vi "main - ONE Motor.vi"() -> ()   [LabVIEW 2018]
uses:
  Ctls/LoggingRate.ctl
  Ctls/MotorConfig.ctl
  Ctls/MotroConfigData.ctl
  Ctls/MagType.ctl
  Ctls/QueueData.ctl
  Ctls/State.ctl
  Ctls/CmdData.ctl
  Ctls/ConsumerLoopData.ctl
  Ctls/DisplayIndicator.ctl
  Ctls/DatabaseCmd.ctl
  Siemens S7 TCP v3_3 LV 8_5/Siemens S7 TCP v3_3 LV 8_5/S7 TCP API Library/S7 TCP.lvlib
panel:
  out "error out":errorcluster
  out "Motor#1_EmoStop?":bool caption="急停指示"
  in  "Speed Setting Checked?_4":bool
  in  "Speed Setting Checked?_3":bool
  in  "Speed Setting Checked?_2":bool
  in  "Speed Setting Checked?_1":bool
  in  "Motor_SpeedSetting#4":dbl caption="电机速度设定 1" min=0.0 max=50.0 format="%.3f"
  in  "Motor_SpeedSetting#3":dbl caption="电机速度设定 1" min=0.0 max=50.0 format="%.3f"
  in  "Motor_SpeedSetting#2":dbl caption="电机速度设定 1" min=0.0 max=50.0 format="%.3f"
  out "Motor#1_Speed":sgl(knob) caption="电机转速RPS" scale=0.01..50.0 scale format="%#.3f"
  out "Motor#1_ConfigData":T1 caption="电机配置数据"
  in  "Motor#1_Config":T2 caption="电机配置"
  in  "Motor#1_SpeedSet?":bool
  in  "Log Length":i32=50
  in  "Logging Rate":T4=enum."5Hz"
  in  "sample interval (ms)":i32=50
  in  "Record":bool
  out "Speed Log to Display":string[][](table)
  out "Data Read":u8[][](array[numeric])
  out "Float Data Valid?":bool[](array[boolean])
  out "Bool Data Valid":bool
  in  "Stop Button":bool
  out "SpeedCurve":sgl(graph) caption="实时显示"
  in  "ClearFault?":bool caption="故障复位"
  out "Motor#1_Fault?":bool caption="故障指示 1"
  out "Motor#1_Running?":bool caption="电机运行指示"
  out "Motor#1_Connected？":bool caption="远程允许"
  out "Motor#1_Current":dbl caption="电机电流   1" format="%1.2f"
  in  "Motor_SpeedSetting#1":dbl caption="电机速度设定 1" min=0.0 max=50.0 format="%.3f"
  in  "Motor#1_Start?":bool caption="电机启动   1"
  in  "Motor#1_Direction":bool caption="电机方向\n正转          反转    1"
  # "1#大电机"
  # "RPS"
  # "RPS"
  # "RPS"
  # "RPS"
  # "A"
  # "注意：切换励磁请手动更改驱动器参数P50082,\n 当P50082=0时为永磁，P50082=1时为励磁！！"
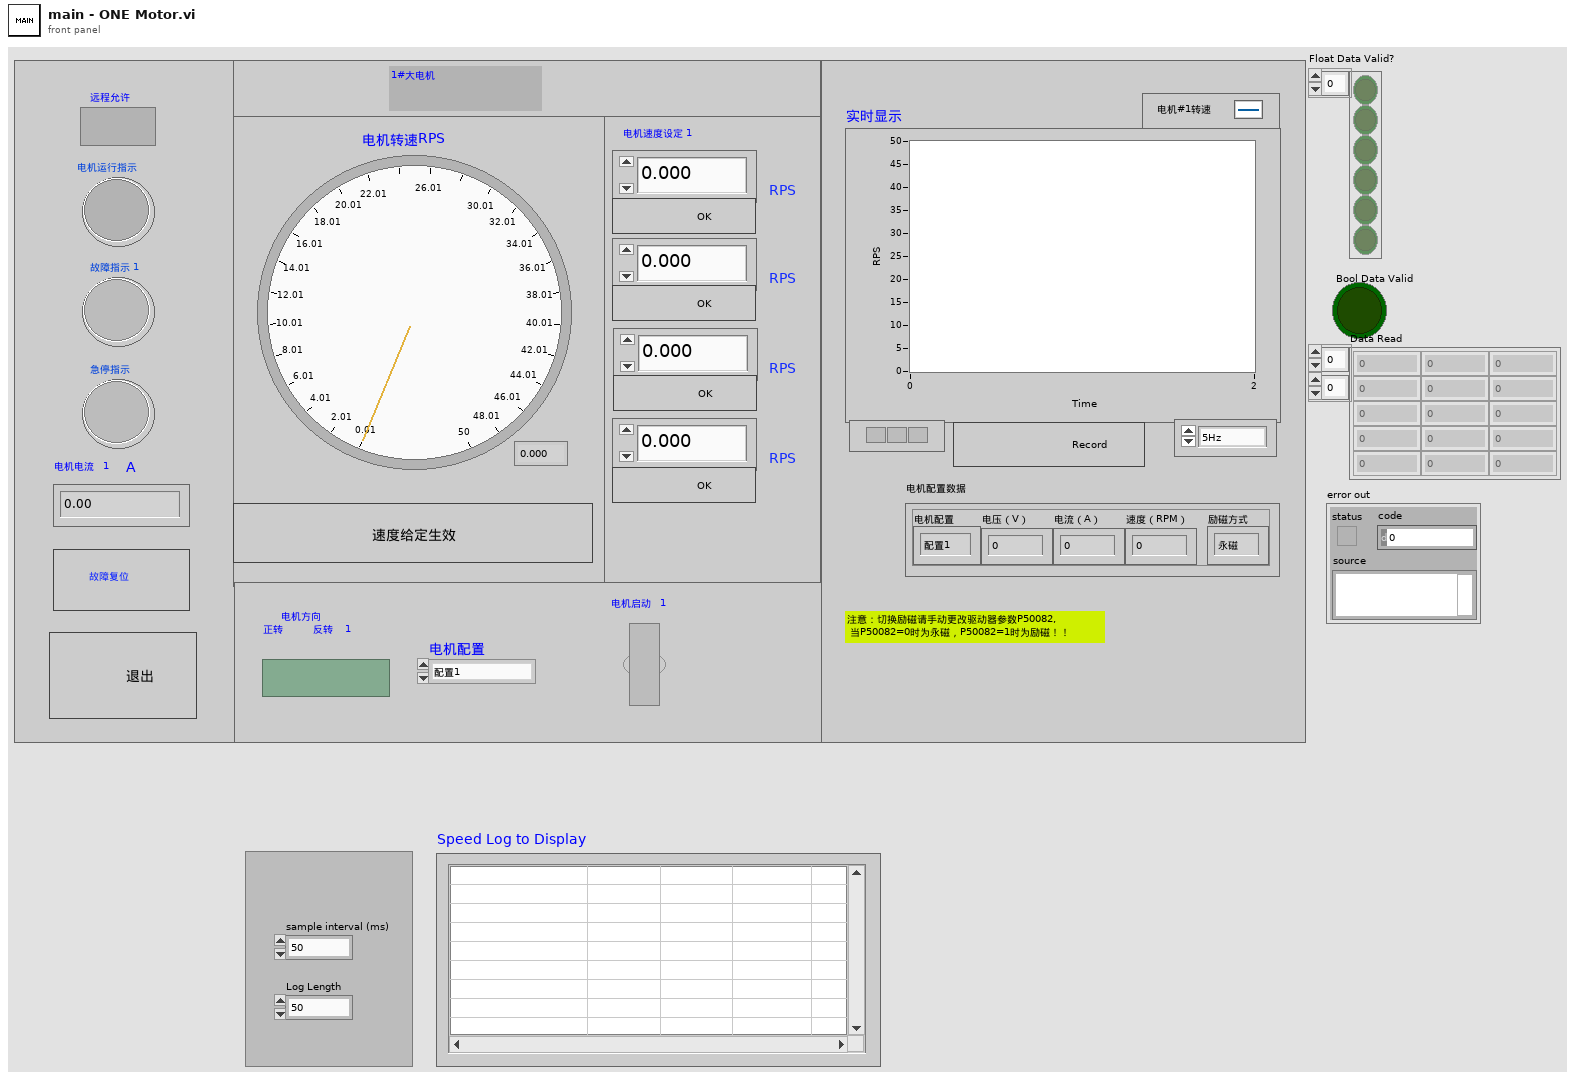
[diagram p1: front panel]
types:
  T1 = typedef "MotroConfigData.ctl" = cluster{"电机配置":T2, "电压（V）":dbl, "电流（A）":dbl, "速度（RPM）":dbl, "励磁方式":T3}
  T2 = typedef "MotorConfig.ctl" = enum16{"配置1", "配置2", "配置3", "配置4"}
  T3 = typedef "MagType.ctl" = enum16{"永磁", "励磁"}
  T4 = typedef "LoggingRate.ctl" = enum16{"1Hz", "2Hz", "5Hz", "10Hz", "20Hz"}
  T5 = typedef "ConsumerLoopData.ctl" = cluster{"CmdU16":u16, "Log File Path":path, "PLC Data":T6, "TCP Connection Ref":refnum<k5>, "Config File Path":path}
  T6 = typedef "DisplayIndicator.ctl" = cluster{"CommConnected_1":bool, "Run_1?":bool, "Fault_1?":bool, "CommConnected_2":bool, "Run_2?":bool, "Fault_2?":bool, "Motor Speed 2":sgl, "Motor Speed_1":sgl, "Motor Current_1":sgl, "Motor Current_2":sgl, "Motor1ConfigData":T1, "Motor2ConfigData":T1, "EmoStop_1?":bool}
  T7 = typedef "State.ctl" = enum16{"poll data command", "display update", "init", "send bool command", "send float command", "datalog", "error", "fix rating rpm 1", "fix rating rpm 2", "fix both rating rpm", "fix rating rpm all", "terminate", "log Motor Speed Setting"}
  T8 = typedef "QueueData.ctl" = cluster{"State":T7, "Command Data":T9}
  T9 = typedef "CmdData.ctl" = cluster{"Address Areas":u8, "Data Block #":u16, "Start Address (bytes)":u32, "Write Data Float":sgl, "Bit #":u16, "Write Data Boolean":bool}
  T10 = typedef "DatabaseCmd.ctl" = enum16{"Insert Table Title", "Add One Record", "Delete Record", "Get Table Records", "Clear"}
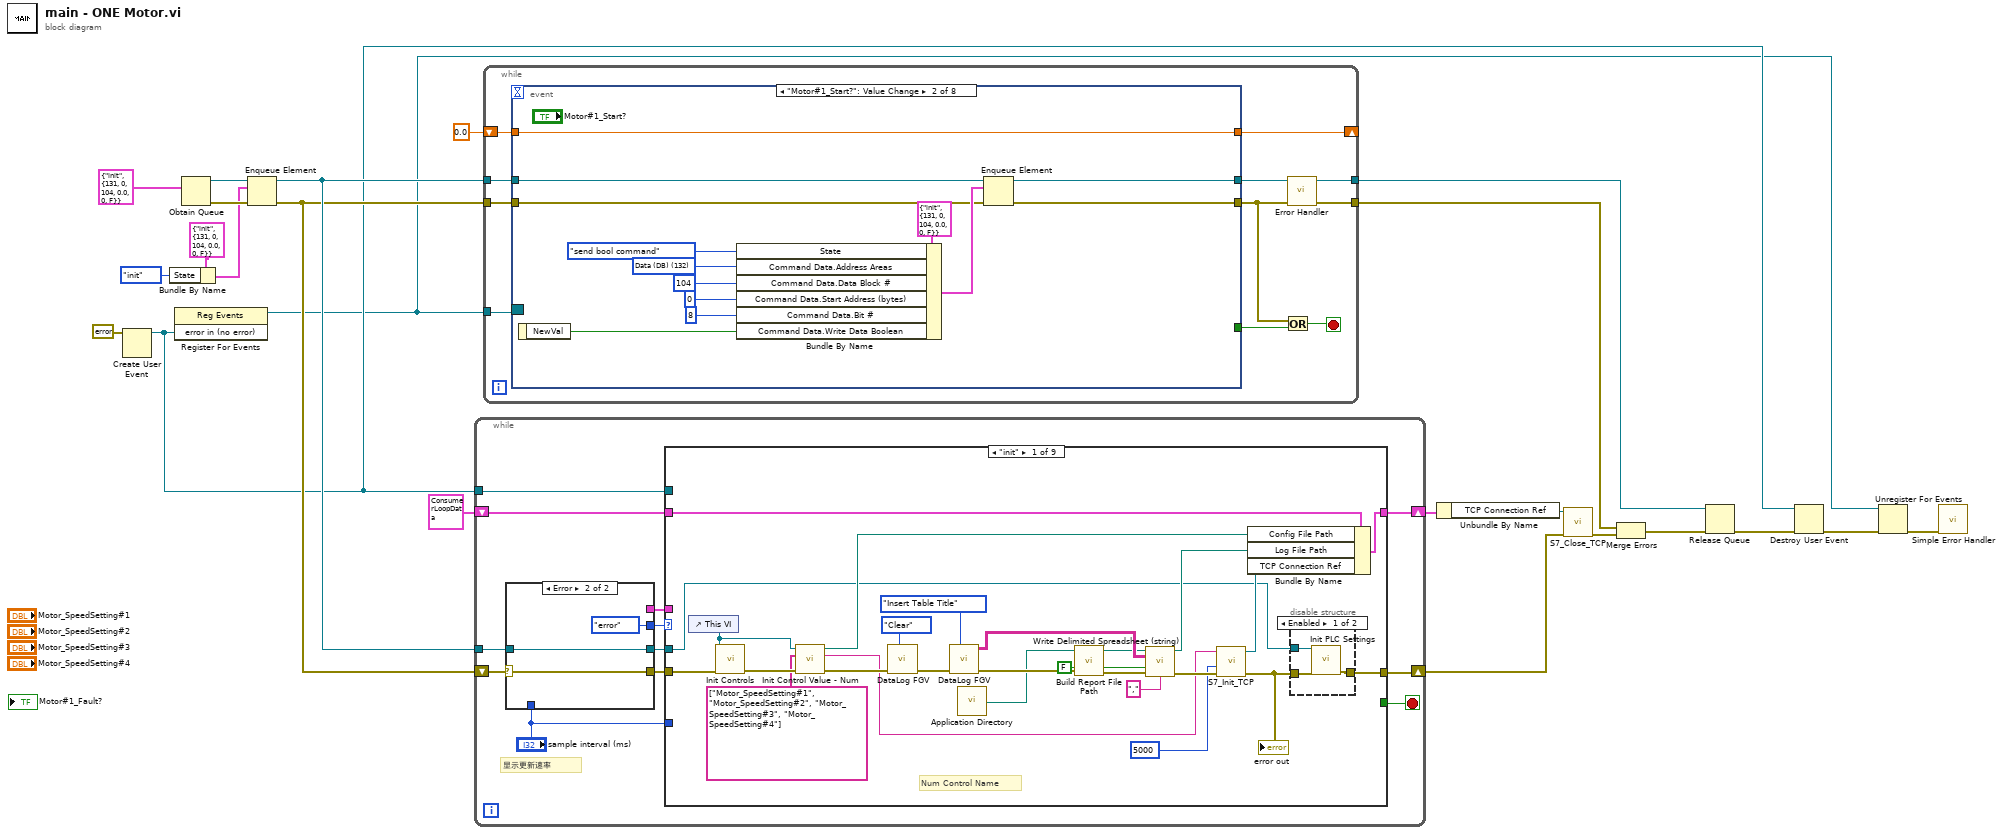
[diagram p0: block diagram]
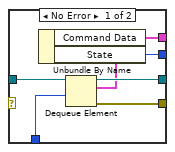
[diagram p2: hidden frame]
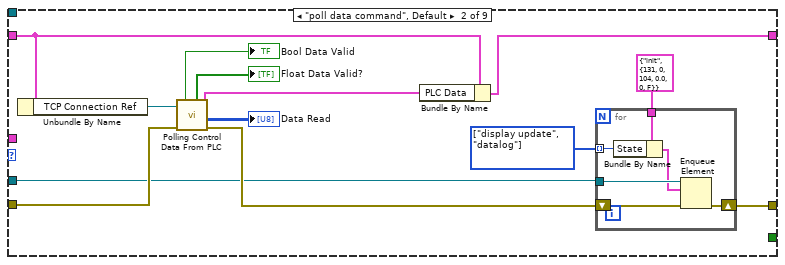
[diagram p4: hidden frame]
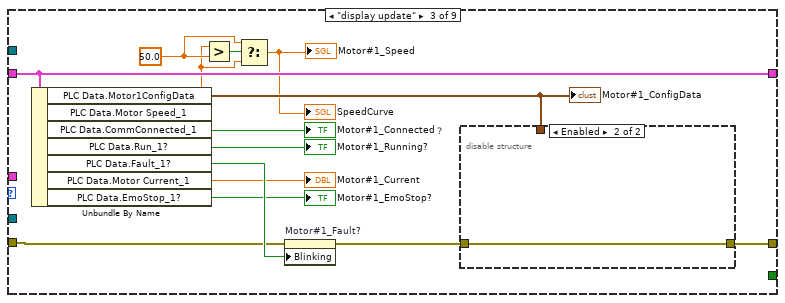
[diagram p5: hidden frame]
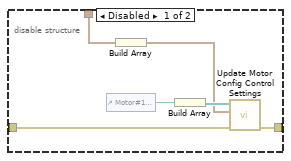
[diagram p6: hidden frame]
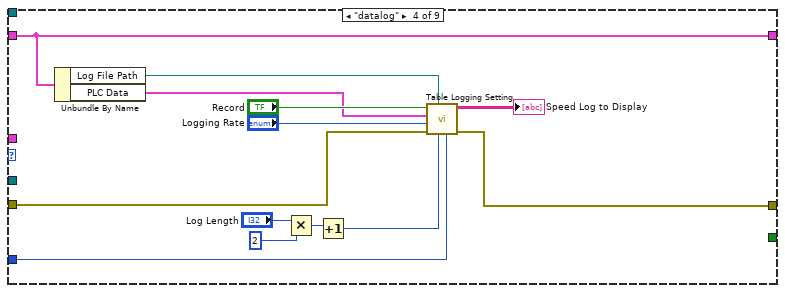
[diagram p7: hidden frame]
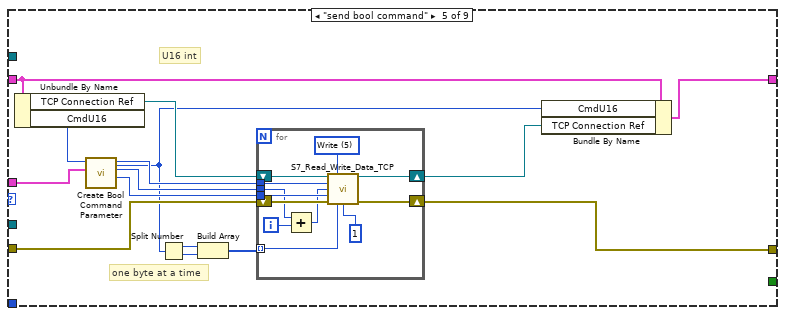
[diagram p8: hidden frame]
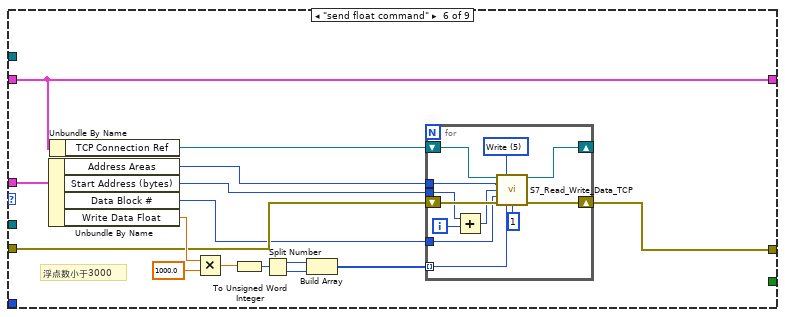
[diagram p9: hidden frame]
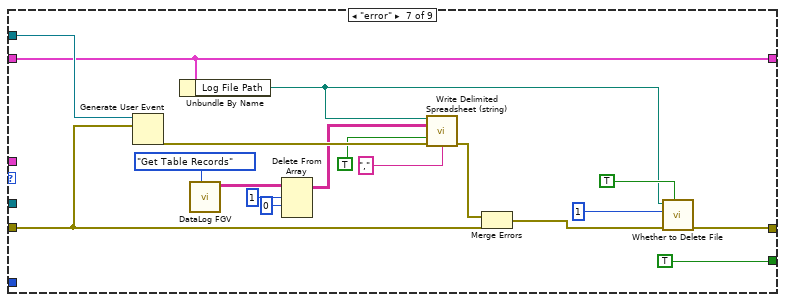
[diagram p10: hidden frame]
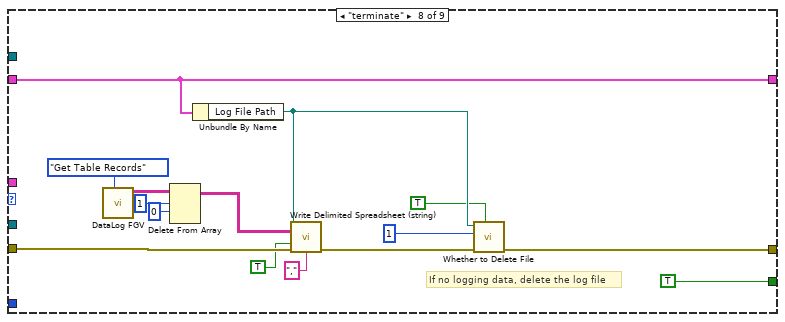
[diagram p11: hidden frame]
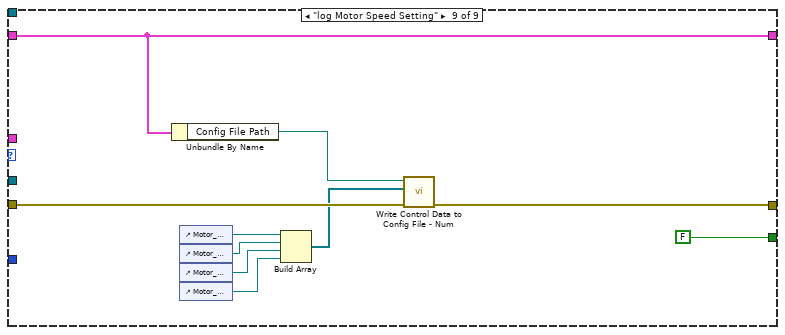
[diagram p12: hidden frame]
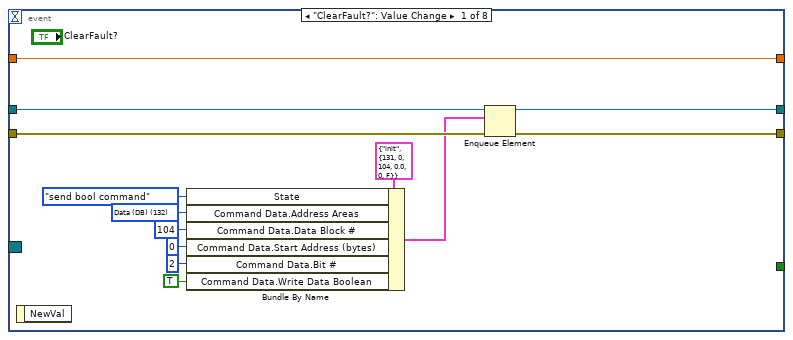
[diagram p13: hidden frame]
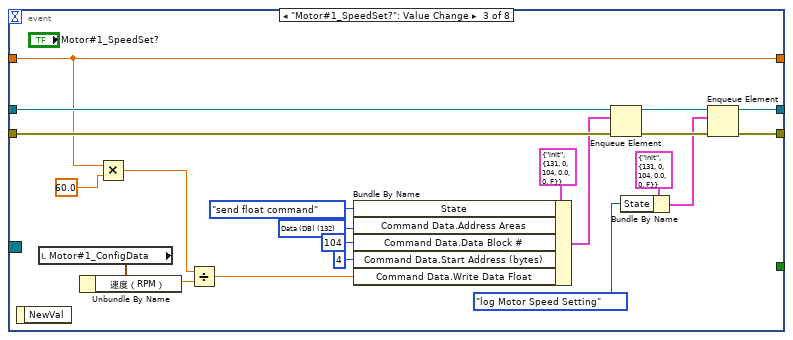
[diagram p14: hidden frame]
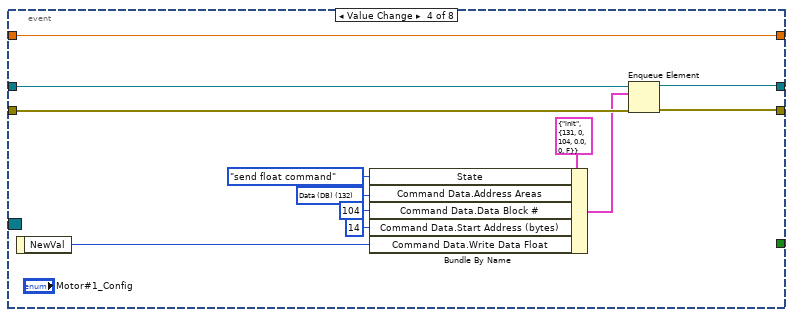
[diagram p15: hidden frame]
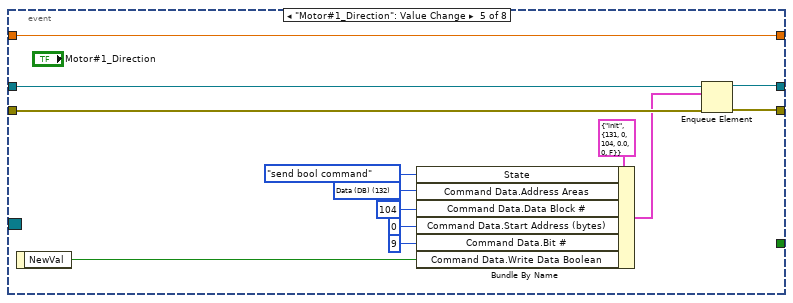
[diagram p16: hidden frame]
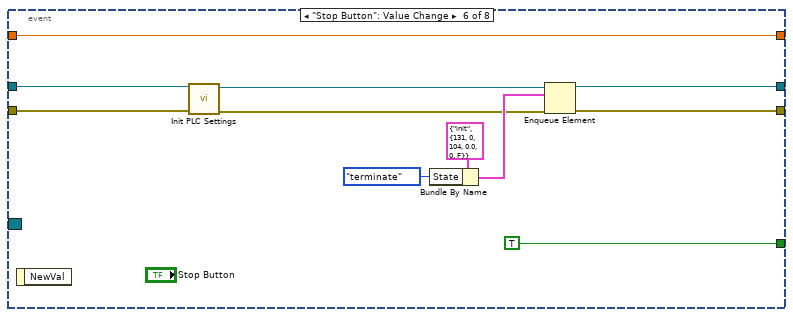
[diagram p17: hidden frame]
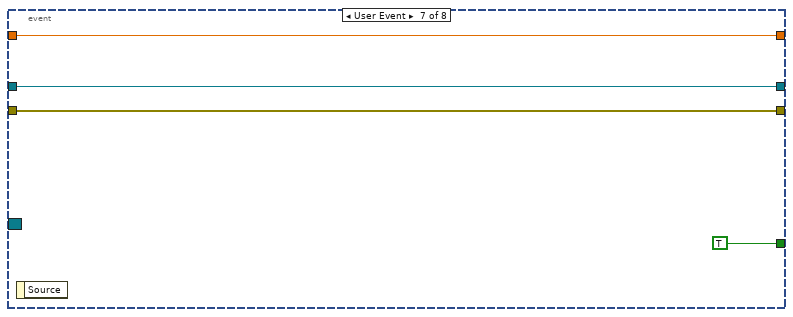
[diagram p18: hidden frame]
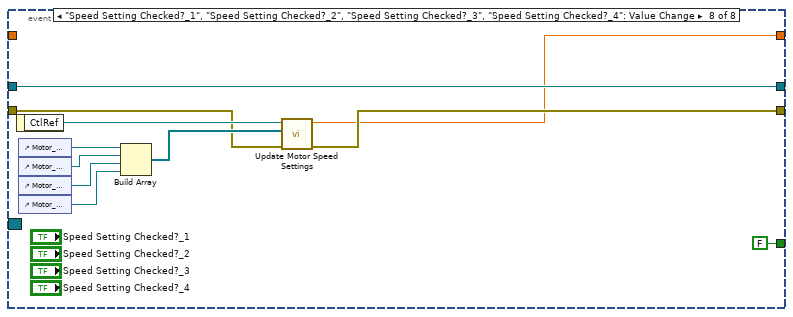
[diagram p19: hidden frame]
diagram:
  n1 = Create User Event(user event datatype=errorcluster {"status"=FALSE, "code"=0, "source"=""} ("error in (no error)")) -> (user event=w14:refnum<user-event>)  [unwired: 1 in, 1 out]
  n2 = Bundle By Name(cluster=T8 {"State"=enum."init", "Command Data"={"Address Areas"=131, "Data Block #"=0, "Start Address (bytes)"=104, "Write Data Float"=0.0, "Bit #"=0, "Write Data Boolean"=FALSE}} ("element"), "State"=State."init") -> (w16:T8)
  n3 = register-events(w14) -> (reference out=w12:refnum<event-registration>)  [unwired: 2 in, 1 out]
  n4 = Obtain Queue(element data type=T8 {"State"=enum."init", "Command Data"={"Address Areas"=131, "Data Block #"=0, "Start Address (bytes)"=104, "Write Data Float"=0.0, "Bit #"=0, "Write Data Boolean"=FALSE}} ("QData")) -> (queue out=w22:refnum<queue>, error out=w20:errorcluster)  [unwired: 4 in, 1 out]
  n5 = Enqueue Element(queue=w22, element=w16, error in (no error)=w20) -> (queue out=w21:refnum<queue>, error out=w19:errorcluster)  [unwired: 1 in, 1 out]
  n6 = while {
    tunnel: w21 -> [w27]
    tunnel: w14 -> [w30]
    shift-right: [w28] -> w11
    shift-left: w19 -> [w29]
    shift-right: [w25] -> w9
    shift-left: T5 {"CmdU16"=0, "Log File Path"=path "", "PLC Data"={"CommConnected_1"=FALSE, "Run_1?"=FALSE, "Fault_1?"=FALSE, "CommConnected_2"=FALSE, "Run_2?"=FALSE, "Fault_2?"=FALSE, "Motor Speed 2"=0.0, "Motor Speed_1"=0.0, "Motor Current_1"=0.0, "Motor Current_2"=0.0, "Motor1ConfigData"={"电机配置"=enum."配置1", "电压（V）"=0.0, "电流（A）"=0.0, "速度（RPM）"=0.0, "励磁方式"=enum."永磁"}, "Motor2ConfigData"={"电机配置"=enum."配置1", "电压（V）"=0.0, "电流（A）"=0.0, "速度（RPM）"=0.0, "励磁方式"=enum."永磁"}, "EmoStop_1?"=FALSE}, "TCP Connection Ref"=refnum, "Config File Path"=path ""} ("Consumer Loop Data") -> [w26]
    stop <- w31 stop-if-true
    # "显示更新速率"
    n7 = case shown="Error" w29 {
      selector: w29 -> [_ w45]
      tunnel: [w42 w44] -> w35
      tunnel: [w41 w45] -> w34
      tunnel: [w39 State."error" ("State")] -> w33
      tunnel: [w38 _] -> w32
      tunnel: w27 -> [w37 w44]
      tunnel: "sample interval (ms)" -> [w36 _]
      frame No Error {
        n8 = Dequeue Element(queue=w37, timeout in ms (-1)=w36) -> (queue out=w42:refnum<queue>, element=w40:T8, error out=w41:errorcluster)  [unwired: 1 in, 1 out]
        n9 = Unbundle By Name(w40) -> ("Command Data"=w38:T9, "State"=w39:T7)
      }
      frame Error {
      }
    }
    n10 = case shown="\"init\"" w33 {
      tunnel: w35 -> [w47 w85 _ _ _ _ _ _ _]
      tunnel: w34 -> [w57 w88 w105 w126 w143 w164 w198 w210 w223]
      tunnel: [w58 w86 w108 w125 w135 w158 w184 w204 w217] -> w28
      tunnel: w32 -> [_ _ _ _ w142 w170 _ _ _]
      tunnel: [_ _ _ _ _ _ TRUE ("Data Valid") TRUE ("Data Valid") FALSE ("Data Valid")] -> w31
      tunnel: w30 -> [_ _ _ _ _ _ w199 _ _]
      tunnel: w26 -> [w56 w82 w107 w117 w132 w156 w188 w206 w225]
      tunnel: [w55 w80 w107 w117 w129 w156 w188 w206 w225] -> w25
      tunnel: "sample interval (ms)" -> [_ _ _ w116 _ _ _ _ _]
      frame "init" {
        # "Num Control Name"
        n11 = control-ref of="This VI"() -> (w48:refnum<vi>)
        n12 = call "Init Controls.vi"("error in"=w57, "VI ref"=w48) -> ("error out"=w54:errorcluster)  [unwired: 9 in]
        n13 = call "Init Control Value - Num.vi"("error in (no error)"=w54, "Num Control Names"=string[] ["Motor_SpeedSetting#1", "Motor_SpeedSetting#2", "Motor_SpeedSetting#3", "Motor_SpeedSetting#4"], "This VI"=w48) -> ("error out"=w53:errorcluster, "PLC IP"=w46:string, "Config File Path"=w50:path)  [unwired: 6 in]
        n14 = call "DataLog FGV.vi"("Method"=DatabaseCmd."Clear", "error in (no error)"=w53) -> ("error out"=w71:errorcluster)  [unwired: 7 in, 2 out]
        n15 = call "DataLog FGV.vi"("Method"=DatabaseCmd."Insert Table Title", "error in (no error)"=w71) -> ("error out"=w70:errorcluster, "Speed Log"=w69:string[][])  [unwired: 7 in, 1 out]
        n16 = call <vilib>:"Application Directory.vi"() -> ("Application Directory"=w63:path)
        n17 = call "Build Report File Path.vi"("error in (no error)"=w70, "File Path in"=w63) -> ("error out"=w67:errorcluster, "Report Path out"=w68:path)  [unwired: 8 in]
        n18 = call "Write Delimited Spreadsheet (string).vi"("Path"=w68, "2D data"=w69, "append to file?"=FALSE ("append to file? (new file:F)"), "error in"=w67, "delimiter (\\t)"="," ("delimiter (\\t)")) -> ("path"=w51:path, "error out"=w61:errorcluster)  [unwired: 9 in]
        n19 = call "S7_Init_TCP.vi"("error in"=w61, "Connection Timeout"=u32 5000, "IP Address"=w46) -> ("error out"=w59:errorcluster, "TCP Connection Ref"=w52:refnum<k5>)  [unwired: 2 in, 5 out]
        "error out" <- w59
        n20 = Bundle By Name(cluster=w56, "Config File Path"=w50, "Log File Path"=w51, "TCP Connection Ref"=w52) -> (w55:T5)
        n21 = disable-structure shown="Enabled" {
          disable-tunnel: w59 -> [w74 w75]
          disable-tunnel: [w73 w75] -> w58
          disable-tunnel: w47 -> [w72 _]
          frame Enabled {
            n22 = call "Init PLC Settings.vi"("error in"=w74, "queue in"=w72) -> ("error out"=w73:errorcluster)  [unwired: 8 in, 1 out]
          }
          frame Disabled {
          }
        }
      }
      frame "poll data command", Default {
        w83 = T7[] [enum."display update", enum."datalog"] items=["poll data command", "display update", "init", "send bool command", "send float command", "datalog", "error", "fix rating rpm 1", "fix rating rpm 2", "fix both rating rpm", "fix rating rpm all", "terminate", "log Motor Speed Setting"]
        n23 = Unbundle By Name(w82) -> ("TCP Connection Ref"=w79:refnum<k5>)
        n24 = call "Polling Control Data From PLC.vi"("error in (no error)"=w88, "TCP Network Connection in"=w79) -> ("error out"=w87:errorcluster, "Data Read"=→"Data Read":u8[][], "PLC Data out"=w81:T6, "Bool Data Valid"=→"Bool Data Valid":bool, "Float Data Valid?"=→"Float Data Valid?":bool[])  [unwired: 2 in, 3 out]
        n25 = Bundle By Name(cluster=w82, "PLC Data"=w81) -> (w80:T5)
        n26 = for {
          tunnel: w85 -> [w92]
          shift-right: [w93] -> w86
          shift-left: w87 -> [w94]
          tunnel: T8 {"State"=enum."init", "Command Data"={"Address Areas"=131, "Data Block #"=0, "Start Address (bytes)"=104, "Write Data Float"=0.0, "Bit #"=0, "Write Data Boolean"=FALSE}} ("QData") -> [w90]
          tunnel: w83 -> [w89] mode=indexing
          n27 = Bundle By Name(cluster=w90, "State"=w89) -> (w91:T8)
          n28 = Enqueue Element(queue=w92, element=w91, error in (no error)=w94) -> (error out=w93:errorcluster)  [unwired: 1 in, 2 out]
        }
      }
      frame "display update" {
        w98 = sgl 50.0 ("y")
        n29 = Unbundle By Name(w107) -> ("PLC Data.Motor1ConfigData"=w100:T1, "PLC Data.Motor Speed_1"=w97:sgl, "PLC Data.CommConnected_1"=→"Motor#1_Connected？":bool, "PLC Data.Run_1?"=→"Motor#1_Running?":bool, "PLC Data.Fault_1?"=w106:bool, "PLC Data.Motor Current_1"=→"Motor#1_Current":sgl, "PLC Data.EmoStop_1?"=→"Motor#1_EmoStop?":bool)
        "Motor#1_ConfigData" <- w100
        n30 = Greater?(x=w97, y=w98) -> (0:w99:bool)
        n31 = Select(t=w98, s=w99, f=w97) -> (s? t:f=→"SpeedCurve" →"Motor#1_Speed":sgl)
        n32 = property on="Motor#1_Fault?" class="Bool (strict)"(error in=w105, "Blinking"=w106) -> (error out=w101:errorcluster)  [unwired: 1 in, 1 out]
        n33 = disable-structure shown="Enabled" {
          disable-tunnel: [w114 w115] -> w108
          disable-tunnel: w101 -> [w113 w115]
          disable-tunnel: w100 -> [w110 _]
          frame Disabled {
            n34 = control-ref of="Motor#1_Config"() -> (w112:refnum<vi>)
            n35 = Build Array(w110) -> (w109:T1[])
            n36 = Build Array(w112) -> (w111:refnum<vi>[])
            n37 = call "Update Motor Config Control Settings.vi"("error in (no error)"=w113, "Motor Config Data"=w109, "Motor Config Refs"=w111) -> ("error out"=w114:errorcluster)  [unwired: 8 in]
          }
          frame Enabled {
          }
        }
      }
      frame "datalog" {
        n38 = Unbundle By Name(w117) -> ("Log File Path"=w119:path, "PLC Data"=w118:T6)
        n39 = Multiply(x="Log Length", y=2) -> (x*y=w121:i32)
        n40 = Increment(x=w121) -> (x+1=w120:i32)
        n41 = call "Table Logging Setting.vi"("sample interval (ms)"=w116, "Log Length"=w120, "Log File path"=w119, "error in (no error)"=w126, "Logging Rate"="Logging Rate", "Data In"=w118, "Record"="Record") -> ("error out"=w125:errorcluster, "Speed Log to Display"=→"Speed Log to Display":string[][])  [unwired: 3 in]
      }
      frame "send bool command" {
        # "one byte at a time"
        # "U16 int"
        n42 = Unbundle By Name(w132) -> ("TCP Connection Ref"=w133:refnum<k5>, "CmdU16"=w134:u16)
        n43 = call "Create Bool Command Parameter.vi"("Command Data"=w142, "Cmd U16"=w134) -> ("Data Block #"=w139:u16, "Start Address (bytes)"=w140:u32, "Address Areas"=w141:u8, "Cmd U16 out"=w131:u16)  [unwired: 6 in]
        n44 = Split Number(x=w131) -> (hi(x)=w137:u8, lo(x)=w136:u8)
        n45 = Build Array(w137, w136) -> (w138:u8[])
        n46 = for {
          tunnel: w141 -> [w151]
          tunnel: w140 -> [w145]
          tunnel: w139 -> [w150]
          shift-right: [w152] -> w130
          shift-left: w133 -> [w155]
          shift-right: [w148] -> w135
          shift-left: w143 -> [w154]
          tunnel: w138 -> [w147] mode=indexing
          i -> [w146]
          w153 = u8 5 items=["Read"=4, "Write"=5] ("Read / Write")
          n47 = Add(x=w145, y=w146) -> (x+y=w144:u32)
          n48 = call "S7_Read_Write_Data_TCP.vi"("TCP Connection Ref"=w155, "Read / Write"=w153, "Address Areas"=w151, "Start Address (bytes)"=w144, "Data Block #"=w150, "error in"=w154, "Write Data"=w147, "Length (bytes)"=u16 1) -> ("TCP Connection Ref Out"=w152:refnum<k5>, "error out"=w148:errorcluster)  [unwired: 2 in, 4 out]
        }
        n49 = Bundle By Name(cluster=w132, "CmdU16"=w131, "TCP Connection Ref"=w130) -> (w129:T5)
      }
      frame "send float command" {
        # "浮点数小于3000"
        n50 = Unbundle By Name(w170) -> ("Address Areas"=w163:u8, "Start Address (bytes)"=w162:u32, "Data Block #"=w161:u16, "Write Data Float"=w169:sgl)
        n51 = Unbundle By Name(w156) -> ("TCP Connection Ref"=w157:refnum<k5>)
        n52 = Multiply(x=w169, y=sgl 1000.0) -> (x*y=w167:sgl)
        n53 = To Unsigned Word Integer(number=w167) -> (unsigned 16bit integer=w166:u16)
        n54 = Split Number(x=w166) -> (hi(x)=w160:u8, lo(x)=w159:u8)
        n55 = Build Array(w160, w159) -> (w165:u8[])
        n56 = for {
          shift-right: [w179] -> _
          shift-left: w157 -> [w182]
          shift-right: [w177] -> w158
          shift-left: w164 -> [w181]
          tunnel: w165 -> [w174] mode=indexing
          tunnel: w163 -> [w173]
          tunnel: w162 -> [w172]
          tunnel: w161 -> [w171]
          i -> [w176]
          w180 = u8 5 items=["Read"=4, "Write"=5] ("Read / Write")
          n57 = Add(x=w172, y=w176) -> (x+y=w175:u32)
          n58 = call "S7_Read_Write_Data_TCP.vi"("TCP Connection Ref"=w182, "Read / Write"=w180, "Address Areas"=w173, "Start Address (bytes)"=w175, "Data Block #"=w171, "error in"=w181, "Write Data"=w174, "Length (bytes)"=u16 1) -> ("TCP Connection Ref Out"=w179:refnum<k5>, "error out"=w177:errorcluster)  [unwired: 2 in, 4 out]
        }
      }
      frame "error" {
        n59 = Generate User Event(user event=w199, event data cluster=w198) -> (error out=w197:errorcluster)  [unwired: 2 in, 1 out]
        n60 = Unbundle By Name(w188) -> ("Log File Path"=w183:path)
        n61 = call "DataLog FGV.vi"("Method"=DatabaseCmd."Get Table Records") -> ("Speed Log"=w193:string[][])  [unwired: 8 in, 2 out]
        n62 = Delete From Array(array=w193, length=1, index (row)=0) -> (array with subset deleted=w190:string[][])  [unwired: 1 in, 1 out]
        n63 = call "Write Delimited Spreadsheet (string).vi"("Path"=w183, "2D data"=w190, "append to file?"=TRUE ("append to file? (new file:F)"), "error in"=w197, "delimiter (\\t)"="," ("delimiter (\\t)")) -> ("error out"=w196:errorcluster)  [unwired: 9 in, 1 out]
        n64 = Merge Errors(w196, w198) -> (w185:errorcluster)
        n65 = call "Whether to Delete File.vi"("Del Log file?"=TRUE, "error in (no error)"=w185, "Number of lines"=1, "File path"=w183) -> ("error out"=w184:errorcluster)  [unwired: 7 in]
      }
      frame "terminate" {
        # "If no logging data, delete the log file"
        n66 = call "DataLog FGV.vi"("Method"=DatabaseCmd."Get Table Records") -> ("Speed Log"=w213:string[][])  [unwired: 8 in, 2 out]
        n67 = Delete From Array(array=w213, length=1, index (row)=0) -> (array with subset deleted=w209:string[][])  [unwired: 1 in, 1 out]
        n68 = Unbundle By Name(w206) -> ("Log File Path"=w203:path)
        n69 = call "Write Delimited Spreadsheet (string).vi"("Path"=w203, "2D data"=w209, "append to file?"=TRUE ("append to file? (new file:F)"), "error in"=w210, "delimiter (\\t)"="," ("delimiter (\\t)")) -> ("error out"=w205:errorcluster)  [unwired: 9 in, 1 out]
        n70 = call "Whether to Delete File.vi"("Del Log file?"=TRUE, "error in (no error)"=w205, "Number of lines"=1, "File path"=w203) -> ("error out"=w204:errorcluster)  [unwired: 7 in]
      }
      frame "log Motor Speed Setting" {
        n71 = Unbundle By Name(w225) -> ("Config File Path"=w224:path)
        n72 = control-ref of="Motor_SpeedSetting#1"() -> (w222:refnum<vi>)
        n73 = control-ref of="Motor_SpeedSetting#2"() -> (w221:refnum<vi>)
        n74 = control-ref of="Motor_SpeedSetting#3"() -> (w220:refnum<vi>)
        n75 = control-ref of="Motor_SpeedSetting#4"() -> (w219:refnum<vi>)
        n76 = Build Array(w222, w221, w220, w219) -> (w218:refnum<vi>[])
        n77 = call "Write Control Data to Config File - Num.vi"("error in (no error)"=w223, "Num Controls"=w218, "Config File Path"=w224) -> ("error out"=w217:errorcluster)  [unwired: 8 in]
      }
    }
  }
  n78 = while {
    tunnel: w21 -> [w236]
    tunnel: w19 -> [w235]
    tunnel: w12 -> [w234]
    tunnel: [w229] -> w6
    tunnel: [w228] -> w5
    shift-right: [w227] -> _
    shift-left: 0.0 ("Motor Speed") -> [w226]
    stop <- w232 stop-if-true
    n79 = event shown="[1] \"Motor#1_Start?\": Value Change" {
      selector: w234 -> [_ _ _ _ _ _ _ _]
      dyn-events: _ -> [_ _ _ _ _ _ _ _]
      timeout: _ -> [_ _ _ _ _ _ _ _]
      tunnel: [_ _ _ _ _ TRUE ("Stop Button") TRUE ("Stop Button") FALSE ("Stop Button")] -> w233
      tunnel: w236 -> [w249 w259 w282 w294 w307 w313 w323 w328]
      tunnel: w235 -> [w248 w258 w281 w292 w305 w311 w322 w327]
      tunnel: [w244 w251 w269 w293 w306 w318 w323 w328] -> w231
      tunnel: [w245 w250 w264 w291 w304 w317 w322 w326] -> w230
      tunnel: [w237 w252 w263 w284 w296 w309 w320 w324] -> w227
      tunnel: w226 -> [w237 w252 w263 w284 w296 w309 w320 _]
      event "ClearFault?": Value Change {
        w242 = u8 132 items=["I/O (P)"=128, "Input (I)"=129, "Output (Q)"=130, "Bit Memory (M)"=131, "Data (DB)"=132, "Instance Data (DI)"=133, "Local Data (L)"=134, "Predecessor Local Data (VL)"=135] ("Address Areas")
        n80 = event-data() -> ()  [unwired: 1 in, 1 out]
        n81 = Bundle By Name(cluster=T8 {"State"=enum."init", "Command Data"={"Address Areas"=131, "Data Block #"=0, "Start Address (bytes)"=104, "Write Data Float"=0.0, "Bit #"=0, "Write Data Boolean"=FALSE}} ("QData"), "State"=State."send bool command", "Command Data.Address Areas"=w242, "Command Data.Data Block #"=u16 104 ("Data Block #"), "Command Data.Start Address (bytes)"=u32 0 ("Start Address (bytes)"), "Command Data.Bit #"=u16 2 ("Bit #"), "Command Data.Write Data Boolean"=TRUE ("Write Data Boolean")) -> (w247:T8)
        n82 = Enqueue Element(queue=w249, element=w247, error in (no error)=w248) -> (queue out=w244:refnum<queue>, error out=w245:errorcluster)  [unwired: 1 in, 1 out]
      }
      event "Motor#1_Start?": Value Change {
        w257 = u8 132 items=["I/O (P)"=128, "Input (I)"=129, "Output (Q)"=130, "Bit Memory (M)"=131, "Data (DB)"=132, "Instance Data (DI)"=133, "Local Data (L)"=134, "Predecessor Local Data (VL)"=135] ("Address Areas")
        n83 = event-data() -> ("NewVal"=w253:bool)  [unwired: 1 in]
        n84 = Bundle By Name(cluster=T8 {"State"=enum."init", "Command Data"={"Address Areas"=131, "Data Block #"=0, "Start Address (bytes)"=104, "Write Data Float"=0.0, "Bit #"=0, "Write Data Boolean"=FALSE}} ("QData"), "State"=State."send bool command", "Command Data.Address Areas"=w257, "Command Data.Data Block #"=u16 104 ("Data Block #"), "Command Data.Start Address (bytes)"=u32 0 ("Start Address (bytes)"), "Command Data.Bit #"=u16 8 ("Bit #"), "Command Data.Write Data Boolean"=w253) -> (w261:T8)
        n85 = Enqueue Element(queue=w259, element=w261, error in (no error)=w258) -> (queue out=w251:refnum<queue>, error out=w250:errorcluster)  [unwired: 1 in, 1 out]
      }
      event "Motor#1_SpeedSet?": Value Change {
        w274 = u8 132 items=["I/O (P)"=128, "Input (I)"=129, "Output (Q)"=130, "Bit Memory (M)"=131, "Data (DB)"=132, "Instance Data (DI)"=133, "Local Data (L)"=134, "Predecessor Local Data (VL)"=135] ("Address Areas")
        n86 = event-data() -> ()  [unwired: 1 in, 1 out]
        n87 = local read "Motor#1_ConfigData"() -> (w276:T1)
        n88 = Unbundle By Name(w276) -> ("速度（RPM）"=w275:dbl)
        n89 = Multiply(x=w263, y=60.0) -> (x*y=w277:dbl)
        n90 = Divide(x=w277, y=w275) -> (x/y=w271:dbl)
        n91 = Bundle By Name(cluster=T8 {"State"=enum."init", "Command Data"={"Address Areas"=131, "Data Block #"=0, "Start Address (bytes)"=104, "Write Data Float"=0.0, "Bit #"=0, "Write Data Boolean"=FALSE}} ("QData"), "State"=State."send float command", "Command Data.Address Areas"=w274, "Command Data.Data Block #"=u16 104 ("Data Block #"), "Command Data.Start Address (bytes)"=u32 4 ("Start Address (bytes)"), "Command Data.Write Data Float"=w271) -> (w280:T8)
        n92 = Enqueue Element(queue=w282, element=w280, error in (no error)=w281) -> (queue out=w270:refnum<queue>, error out=w268:errorcluster)  [unwired: 1 in, 1 out]
        n93 = Bundle By Name(cluster=T8 {"State"=enum."init", "Command Data"={"Address Areas"=131, "Data Block #"=0, "Start Address (bytes)"=104, "Write Data Float"=0.0, "Bit #"=0, "Write Data Boolean"=FALSE}} ("QData"), "State"=State."log Motor Speed Setting") -> (w265:T8)
        n94 = Enqueue Element(queue=w270, element=w265, error in (no error)=w268) -> (queue out=w269:refnum<queue>, error out=w264:errorcluster)  [unwired: 1 in, 1 out]
      }
      event Value Change {
        w288 = u8 132 items=["I/O (P)"=128, "Input (I)"=129, "Output (Q)"=130, "Bit Memory (M)"=131, "Data (DB)"=132, "Instance Data (DI)"=133, "Local Data (L)"=134, "Predecessor Local Data (VL)"=135] ("Address Areas")
        n95 = event-data() -> ("NewVal"=w285:T2)  [unwired: 1 in]
        n96 = Bundle By Name(cluster=T8 {"State"=enum."init", "Command Data"={"Address Areas"=131, "Data Block #"=0, "Start Address (bytes)"=104, "Write Data Float"=0.0, "Bit #"=0, "Write Data Boolean"=FALSE}} ("QData"), "State"=State."send float command", "Command Data.Address Areas"=w288, "Command Data.Data Block #"=u16 104 ("Data Block #"), "Command Data.Start Address (bytes)"=u32 14 ("Start Address (bytes)"), "Command Data.Write Data Float"=w285) -> (w290:T8)
        n97 = Enqueue Element(queue=w294, element=w290, error in (no error)=w292) -> (queue out=w293:refnum<queue>, error out=w291:errorcluster)  [unwired: 1 in, 1 out]
      }
      event "Motor#1_Direction": Value Change {
        w301 = u8 132 items=["I/O (P)"=128, "Input (I)"=129, "Output (Q)"=130, "Bit Memory (M)"=131, "Data (DB)"=132, "Instance Data (DI)"=133, "Local Data (L)"=134, "Predecessor Local Data (VL)"=135] ("Address Areas")
        n98 = event-data() -> ("NewVal"=w297:bool)  [unwired: 1 in]
        n99 = Bundle By Name(cluster=T8 {"State"=enum."init", "Command Data"={"Address Areas"=131, "Data Block #"=0, "Start Address (bytes)"=104, "Write Data Float"=0.0, "Bit #"=0, "Write Data Boolean"=FALSE}} ("QData"), "State"=State."send bool command", "Command Data.Address Areas"=w301, "Command Data.Data Block #"=u16 104 ("Data Block #"), "Command Data.Start Address (bytes)"=u32 0 ("Start Address (bytes)"), "Command Data.Bit #"=u16 9 ("Bit #"), "Command Data.Write Data Boolean"=w297) -> (w303:T8)
        n100 = Enqueue Element(queue=w307, element=w303, error in (no error)=w305) -> (queue out=w306:refnum<queue>, error out=w304:errorcluster)  [unwired: 1 in, 1 out]
      }
      event "Stop Button": Value Change {
        n101 = event-data() -> ()  [unwired: 1 in, 1 out]
        n102 = call "Init PLC Settings.vi"("error in"=w311, "queue in"=w313) -> ("error out"=w310:errorcluster, "queue out"=w312:refnum<queue>)  [unwired: 8 in]
        n103 = Bundle By Name(cluster=T8 {"State"=enum."init", "Command Data"={"Address Areas"=131, "Data Block #"=0, "Start Address (bytes)"=104, "Write Data Float"=0.0, "Bit #"=0, "Write Data Boolean"=FALSE}} ("QData"), "State"=State."terminate") -> (w315:T8)
        n104 = Enqueue Element(queue=w312, element=w315, error in (no error)=w310) -> (queue out=w318:refnum<queue>, error out=w317:errorcluster)  [unwired: 1 in, 1 out]
      }
      event User Event {
        n105 = event-data() -> ()  [unwired: 1 in, 1 out]
      }
      event "Speed Setting Checked?_1", "Speed Setting Checked?_2", "Speed Setting Checked?_3", "Speed Setting Checked?_4": Value Change {
        n106 = event-data() -> ("CtlRef"=w330:refnum<vi>)  [unwired: 1 in]
        n107 = control-ref of="Motor_SpeedSetting#1"() -> (w334:refnum<vi>)
        n108 = control-ref of="Motor_SpeedSetting#2"() -> (w333:refnum<vi>)
        n109 = control-ref of="Motor_SpeedSetting#3"() -> (w332:refnum<vi>)
        n110 = control-ref of="Motor_SpeedSetting#4"() -> (w331:refnum<vi>)
        n111 = Build Array(w334, w333, w332, w331) -> (w329:refnum<vi>[])
        n112 = call "Update Motor Speed Settings.vi"("error in (no error)"=w327, "Motor_Speed Setting Ref Array"=w329, "Bool RefIn"=w330) -> ("error out"=w326:errorcluster, "Motor Speed"=w324:dbl)  [unwired: 7 in]
      }
    }
    n113 = Or(x=w230, y=w233) -> (x .or. y?=w232:bool)
    n114 = call "Error Handler.vi"("error in (no error)"=w230, "queue in"=w231) -> ("error out"=w229:errorcluster, "queue out"=w228:refnum<queue>)  [unwired: 8 in]
  }
  n115 = Unbundle By Name(w9) -> ("TCP Connection Ref"=w8:refnum<k5>)
  n116 = call "S7_Close_TCP.vi"("error in"=w11, "TCP Connection Ref"=w8) -> ("error out"=w7:errorcluster)  [unwired: 1 in, 8 out]
  n117 = Merge Errors(w6, w7) -> (w4:errorcluster)
  n118 = Release Queue(queue=w5, error in (no error)=w4) -> (error out=w3:errorcluster)  [unwired: 1 in, 2 out]
  n119 = Destroy User Event(user event=w14, error in=w3) -> (error out=w13:errorcluster)
  n120 = Unregister For Events(event registration refnum=w12, error in=w13) -> (error out=w2:errorcluster)
  n121 = call <vilib>:"Simple Error Handler.vi"("error in (no error)"=w2) -> ()  [unwired: 4 in, 5 out]
